vi "Result_Test.vi"(8 "error in (no error)":errorcluster caption="entrée d'erreur (pas d'erreur)", 11 "Delay en entrée":refnum<class "P1833_Scan_QRCode.lvclass">) -> (0 "error out":errorcluster caption="sortie d'erreur", 3 "Delay en sortie":refnum<class "P1833_Scan_QRCode.lvclass">)   [LabVIEW 2020, in "Library Test.lvlib" / "P1833_Scan_QRCode.lvclass"]
uses:
  P1833_Scan_QRCode.lvclass
  C:/Users/ngarcin/OneDrive - Altyor/Standard TB/Suite TB45/Class/Test/Test (Default)/Test (Default).lvclass
  Commun VI/TypeDef/Variable Printable.ctl
  Test_Without_Instr/Test_Without_Inst.lvclass
  Commun VI/Library Commun.lvlib
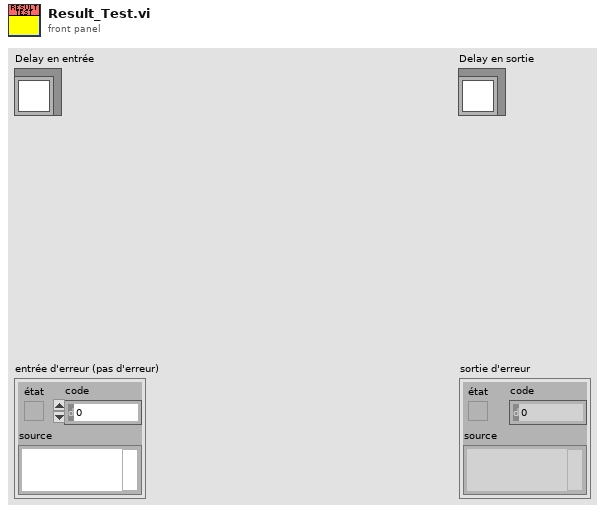
[diagram p1: front panel]
types:
  T1 = enum16{"Get Variable", "Get All Variables", "Set Variable", "Delete Variable", "Delete All Variable"}
  T2 = typedef "Variable Printable.ctl" = string
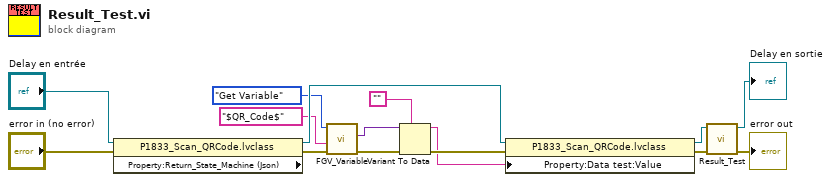
[diagram p0: block diagram]
diagram:
  n1 = property class="P1833_Scan_QRCode.lvclass" props=["Property:Return_State_Machine (Json)"](reference="Delay en entrée", error in="error in (no error)") -> (reference out=w12:refnum<class "P1833_Scan_QRCode.lvclass">, error out=w9:errorcluster)  [unwired: 1 out]
  n2 = call "FGV_Variable.vi"("error in (no error)"=w9, "Variable"=T2 "$QR_Code$", "Function"=T1."Get Variable") -> ("error out"=w6:errorcluster, "Data Out"=w3:variant)  [unwired: 6 in, 1 out]
  n3 = Variant To Data(error in=w6, type="", Variant=w3) -> (data=w2:string, error out=w5:errorcluster)
  n4 = property class="P1833_Scan_QRCode.lvclass"(reference=w12, error in=w5, "Property:Data test:Value"=w2) -> (reference out=w7:refnum<class "P1833_Scan_QRCode.lvclass">, error out=w8:errorcluster)
  n5 = call-parent "Result_Test.vi"("error in (no error)"=w8, "Test_Without_Inst en entrée"=w7) -> ("error out"=→"error out":errorcluster, "Test_Without_Inst en sortie"=→"Delay en sortie":refnum<class "P1833_Scan_QRCode.lvclass">)  [unwired: 8 in]
